vi "_Find Sheet.vi"(8 "error in":errorcluster, 10 "SheetName":string, 11 "SpreadsheetDocument in":refnum<k24>) -> (0 "error out":errorcluster, 2 "Sheet":refnum<k24>, 3 "SpreadsheetDocument out":refnum<k24>)   [LabVIEW 2021, in "Open Xml.lvlib"]
uses:
  Open Xml.lvlib
  D:/git/Open-Xml-LabVIEW/dll/DocumentFormat.OpenXml.dll
  dll/DocumentFormat.OpenXml.dll
  D:/git/Open-Xml-LabVIEW/dll/DocumentFormat.OpenXml.Framework.dll
  dll/DocumentFormat.OpenXml.Framework.dll
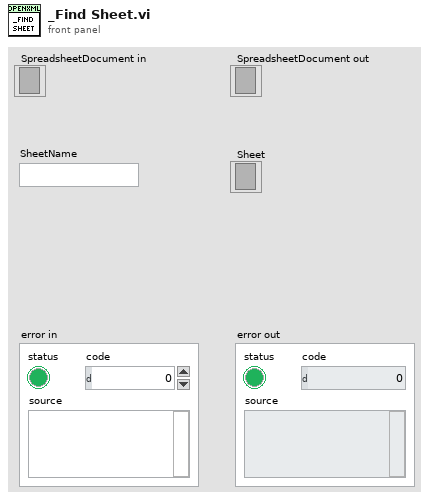
[diagram p1: front panel]
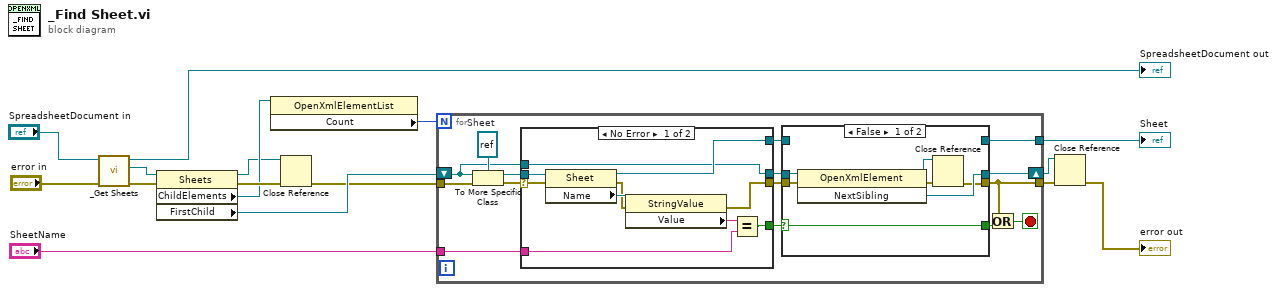
[diagram p0: block diagram]
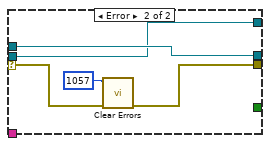
[diagram p3: hidden frame]
diagram:
  n1 = call "_Get Sheets.vi"("error in"="error in", "SpreadsheetDocument in"="SpreadsheetDocument in") -> ("error out"=w9:errorcluster, "Sheets"=w10:refnum<k24>, "SpreadsheetDocument out"=→"SpreadsheetDocument out":refnum<k24>)  [unwired: 7 in]
  n2 = property class="Sheets"(reference=w10, error in=w9) -> (reference out=w5:refnum<k24>, error out=w16:errorcluster, "ChildElements"=w14:refnum<k24>, "FirstChild"=w15:refnum<k24>)
  n3 = property class="OpenXmlElementList"(reference=w14) -> ("Count"=w13:i32)  [unwired: 1 in, 2 out]
  n4 = Close Reference(reference=w5, error in (no error)=w16) -> (error out=w6:errorcluster)
  n5 = for {
    N: w13 -> [_]
    tunnel: w6 -> [w30]
    tunnel: [w18] -> w3
    shift-right: [w23] -> w1
    shift-left: w15 -> [w27]
    tunnel: "SheetName" -> [w25]
    tunnel: [w17] -> w4
    stop <- w19 stop-if-true
    w31 = refnum<k24> refnum  # Sheet
    n6 = To More Specific Class(target class=w31, reference=w27, error in=w30) -> (specific class reference=w26:refnum<k24>, error out=w29:errorcluster)
    n7 = case shown="No Error" w29 {
      selector: w29 -> [w51 w56]
      tunnel: [w44 w55] -> w24
      tunnel: [w42 w53] -> w28
      tunnel: w27 -> [w44 w55]
      tunnel: w26 -> [w50 w54]
      tunnel: w25 -> [w47 _]
      tunnel: [w46 _] -> w21
      tunnel: [w45 w54] -> w22
      frame No Error {
        n8 = property class="Sheet"(reference=w50, error in=w51) -> (reference out=w45:refnum<k24>, error out=w43:errorcluster, "Name"=w49:refnum<k24>)
        n9 = property class="StringValue"(reference=w49, error in=w43) -> (error out=w42:errorcluster, "Value"=w48:string)  [unwired: 1 out]
        n10 = Equal?(x=w48, y=w47) -> (x = y?=w46:bool)
      }
      frame Error {
        n11 = call <vilib>:"Clear Errors.vi"("error in (no error)"=w56, "specific error code to clear (0: all)"=1057) -> ("error out"=w53:errorcluster)  [unwired: 4 in, 1 out]
      }
    }
    n12 = case shown="False" w21 {
      selector: w21 -> [w35 w41]
      tunnel: w28 -> [w38 w40]
      tunnel: [w32 w40] -> w18
      tunnel: w24 -> [w37 _]
      tunnel: [w36 _] -> w23
      tunnel: w22 -> [_ w39]
      tunnel: [w35 w41] -> w20
      tunnel: [_ w39] -> w17
      frame False {
        n13 = invoke class="OpenXmlElement" method="NextSibling"(reference=w37, error in=w38) -> (reference out=w34:refnum<k24>, error out=w33:errorcluster, "NextSibling"=w36:refnum<k24>)  [unwired: 1 in]
        n14 = Close Reference(reference=w34, error in (no error)=w33) -> (error out=w32:errorcluster)
      }
      frame True {
      }
    }
    n15 = Or(x=w18, y=w20) -> (x .or. y?=w19:bool)
  }
  "Sheet" <- w4
  n16 = Close Reference(reference=w1, error in (no error)=w3) -> (error out=→"error out":errorcluster)
